vi "Configure Output Impedance.vi"(6 "Source Impedance (50.0 Ohms)":dbl(ring) items=["50.0", "5.0"], 8 "error in (no error)":errorcluster, 9 "Impedance (50.0 Ohms)":dbl, 10 "Channel (1: Channel1)":u16(ring) items=["Channel1", "Channel2"], 11 "VISA resource name":refnum<visa-resource-name>) -> (0 "error out":errorcluster, 3 "VISA resource name out":refnum<visa-resource-name>)   [LabVIEW 2009, in "Agilent 81150.lvlib"]
doc: "Configures the output impedance and source impedance for the channel you specify."
uses:
  Agilent 81150.lvlib
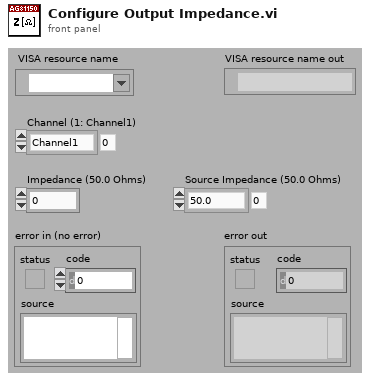
[diagram p1: front panel]
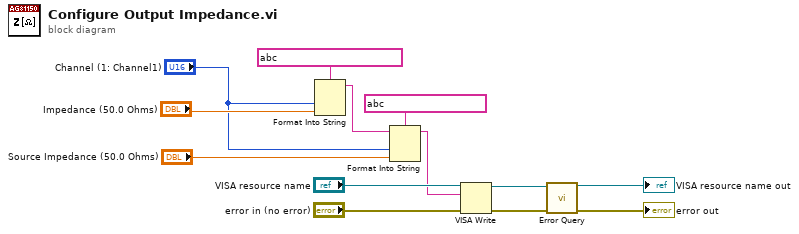
[diagram p0: block diagram]
diagram:
  n1 = Format Into String(format string=string ?, "Channel (1: Channel1)", "Impedance (50.0 Ohms)") -> (resulting string=w4:string)  [unwired: 2 in, 1 out]
  n2 = Format Into String(format string=string ?, initial string=w4, "Channel (1: Channel1)", "Source Impedance (50.0 Ohms)") -> (resulting string=w3:string)  [unwired: 1 in, 1 out]
  n3 = VISA Write(VISA resource name="VISA resource name", write buffer=w3, error in (no error)="error in (no error)") -> (VISA resource name out=w9:refnum<visa-resource-name>, error out=w8:errorcluster)  [unwired: 1 out]
  n4 = call "Error Query.vi"("error in (no error)"=w8, "VISA resource name"=w9) -> ("error out"=→"error out":errorcluster, "VISA resource name out"=→"VISA resource name out":refnum<visa-resource-name>)  [unwired: 8 out]
